vi "Write timer fd.vi"(8 "error in (no error)":errorcluster, 10 "timer fd":i32, 11 "Unix Pipe Reader in":refnum<class "Unix Pipe Reader.lvclass">) -> (0 "error out":errorcluster, 3 "Unix Pipe Reader out":refnum<class "Unix Pipe Reader.lvclass">)   [LabVIEW 2013, in "Linux RT IPC.Pipes.lvlib" / "Unix Pipe Reader.lvclass"]
uses:
  Unix Pipe Reader.lvclass
  Unix Pipe Reader.lvclass/Unix Pipe Reader.ctl
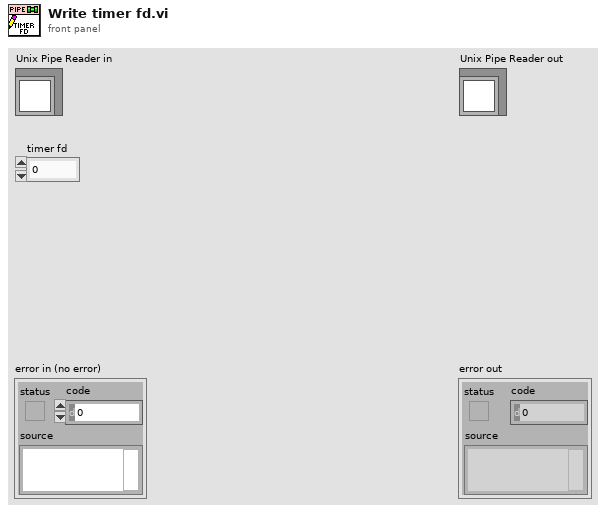
[diagram p1: front panel]
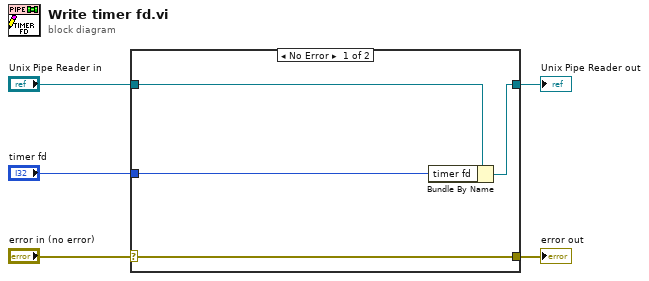
[diagram p0: block diagram]
diagram:
  n1 = case shown="No Error" "error in (no error)" {
    selector: "error in (no error)" -> [w9 w10]
    tunnel: [w9 w10] -> w4
    tunnel: [w7 w11] -> w2
    tunnel: "Unix Pipe Reader in" -> [w8 w11]
    tunnel: "timer fd" -> [w6 _]
    frame No Error {
      n2 = Bundle By Name(cluster=w8, "timer fd"=w6) -> (w7:refnum<class "Unix Pipe Reader.lvclass">)
    }
    frame Error {
    }
  }
  "error out" <- w4
  "Unix Pipe Reader out" <- w2
